vi "TwoCameraDisplayPanel.vi"() -> ()   [LabVIEW 2011]
uses:
  MvLVLib/MvCameraControl.lvlib
  MvLVLib/VIs/CreateGigEHandle.vi
  MvLVLib/VIs/CreateU3VHandle.vi
  <vilib>/picture/picture.llb/imagedata.ctl
panel:
  in  "image data 2":T1 caption="图像数据"
  in  "Rectangle 2":T2
  out "pFrameInfoEx out 2":T3
  in  "pConvertInfo In 2":T4
  out "nWidth 2":u32
  out "nHeight 2":u32
  out "PayloadSize 2":u32
  out "PixelFormat 2":u32
  out "handle out 2":u64
  in  "handle 2":u64
  out "Picture 2":picture
  in  "Device List 2":u16(ring)
  out "U3VDeviceArray":T5(array[cluster])
  out "GigEDeviceArray":T6(array[cluster])
  in  "pConvertInfo In":T4
  out "PixelFormat":u32
  out "handle out":u64
  in  "handle":u64
  in  "Rectangle":T2
  in  "image data":T1 caption="图像数据"
  out "Picture":picture
  out "PayloadSize":u32
  out "pFrameInfoEx out":T3
  out "nHeight":u32
  out "nWidth":u32
  out "Acquisision Flag":bool
  in  "Trigger Mode":bool
  in  "Continuous":bool
  out "打开标志":bool
  in  "stop":bool
  in  "Trigger Once":bool
  in  "Stop":bool
  in  "Start":bool
  in  "Open Device":bool
  in  "Close Device":bool
  in  "error in (no error) 2":errorcluster caption="错误输入（无错误）"
  in  "Refresh Devices":bool
  in  "Device List":u16(ring)
  # "Initialize"
  # "Acquisition"
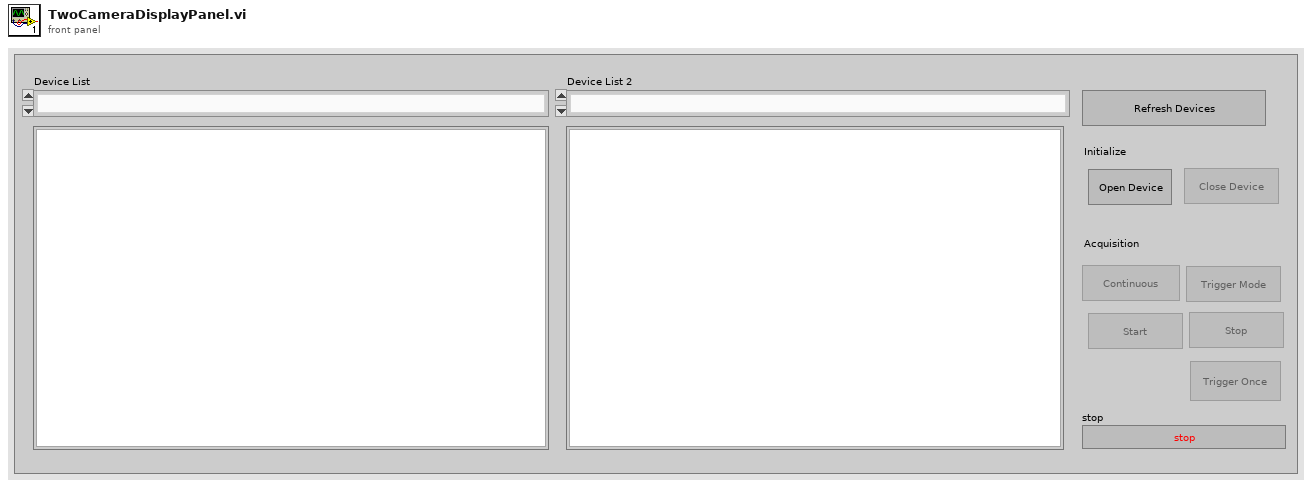
[diagram p1: front panel]
types:
  T1 = typedef "imagedata.ctl" = cluster{"image type":i32, "image depth":i32, "image":u8[], "mask":u8[], "colors":u32[], "Rectangle":cluster{"left":i16, "top":i16, "right":i16, "bottom":i16}}
  T2 = cluster{"left":i16, "top":i16, "right":i16, "bottom":i16}
  T3 = cluster{"nWidth":u16, "nHeight":u16, "enPixelType":i32, "nFrameNum":u32, "nDevTimeStampHigh":u32, "nDevTimeStampLow":u32, "nReserved0":u32, "nHostTimeStamp":i64, "nFrameLen":u32, "nSecondCount]":u32, "nCycleCount":u32, "nCycleOffset":u32, "fGain":u32, "fExposureTime":u32, "nAverageBrightness":u32, "nRed":u32, "nGreen":u32, "nBlue":u32, "nFrameCounter":u32, "nTriggerIndex":u32, "nInput":u32, "nOutput":u32, "nOffsetX":u32, "nOffsetY":u32, "nReserved[0]":u32, "nReserved[1]":u32, "nReserved[2]":u32, "nReserved[3]":u32, "nReserved[4]":u32, "nReserved[5]":u32, "nReserved[6]":u32, "nReserved[7]":u32, "nReserved[8]":u32, "nReserved[9]":u32, "nReserved[10]":u32, "nReserved[11]":u32, "nReserved[12]":u32, "nReserved[13]":u32, "nReserved[14] 10":u32, "nReserved[15] 11":u32, "nReserved[16] 12":u32, "nReserved[17] 13":u32, "nReserved[18] 14":u32, "nReserved[19] 15":u32, "nReserved[20] 16":u32, "nReserved[21] 17":u32, "nReserved[22] 18":u32, "nReserved[23] 19":u32, "nReserved[24] 20":u32, "nReserved[25] 21":u32, "nReserved[26] 22":u32, "nReserved[27] 23":u32, "nReserved[28] 24":u32, "nReserved[29] 25":u32, "nReserved[30] 26":u32, "nReserved[31] 27":u32, "nReserved[32] 28":u32, "nReserved[33] 29":u32, "nReserved[34] 30":u32, "nReserved[35] 31":u32, "nReserved[36] 32":u32, "nReserved[37] 33":u32, "nReserved[38] 34":u32, "nReserved[39] 35":u32, "nReserved[40] 36":u32}
  T4 = cluster{"nWidth":u16, "nHeight":u16, "enSrcPixelType":u32, "nSrcDataLen":u32, "enDstPixelType":u32, "nDstLen":u32, "nDstBufferSize":u32, "nRes0":u32, "nRes1":u32, "nRes2":u32, "nRes3":u32}
  T5 = cluster{"nMajorVer":u16, "nMinorVer":u16, "nMacAddrHigh":u32, "nMacAddrLow":u32, "nTLayerType":u32, "nReserved0":u32, "nReserved1":u32, "nReserved2":u32, "nReserved3":u32, "CrtlInEndPoint":u8, "CrtlOutEndPoint":u8, "StreamEndPoint":u8, "EventEndPoint":u8, "idVendor":u16, "idProduct":u16, "nDeviceNumber":u32, "nRes0":u32, "nRes1":u32, "chDeviceGUID":string, "chVendorName":string, "chModelName":string, "chFamilyName":string, "chDeviceVersion":string, "chManufacturerName":string, "chSerialNumber":string, "chUserDefinedName":string, "nbcdUSB":u32, "nRes2":u32, "nRes3":u32}[]
  T6 = cluster{"nMajorVer":u16, "nMinorVer":u16, "nMacAddrHigh":u32, "nMacAddrLow":u32, "nTLayerType":u32, "nReserved0":u32, "nReserved1":u32, "nReserved2":u32, "nReserved3":u32, "nIpCfgOption":u32, "nIpCfgCurrent":u32, "nCurrentIp":u32, "nCurrentSubNetMask":u32, "nDefaultGateWay":u32, "chManualfacturerName":string, "chModelName":string, "chDeviceVersion":string, "chManufacturerSpecificInfo":string, "chSerialNumber":string, "chUserDefinedName":string, "nRes0":string, "nRes1":string, "nNetExport":u32, "nRes2":u32, "nRes3":u32}[]
  T7 = enum8{"Enabled", "Disabled", "Disabled and Grayed Out"}
  T8 = cluster{"nCurValue":u32, "nMax":u32, "nMin":u32, "nInc":u32, "nReserved[0]":u32, "nReserved[1]":u32, "nReserved[2]":u32, "nReserved[3]":u32}
  T9 = cluster{"nCurValue":u32, "nSupportedNum":u32, "nSupportValue[0]":u32, "nSupportValue[1]":u32, "nSupportValue[2]":u32, "nSupportValue[3]":u32, "nSupportValue[4]":u32, "nSupportValue[5]":u32, "nSupportValue[6]":u32, "nSupportValue[7]":u32, "nSupportValue[8]":u32, "nSupportValue[9]":u32, "nSupportValue[10]":u32, "nSupportValue[11]":u32, "nSupportValue[12]":u32, "nSupportValue[13]":u32, "nSupportValue[14]":u32, "nSupportValue[15]":u32, "nSupportValue[16]":u32, "nSupportValue[17]":u32, "nSupportValue[18]":u32, "nSupportValue[19]":u32, "nSupportValue[20]":u32, "nSupportValue[21]":u32, "nSupportValue[22]":u32, "nSupportValue[23]":u32, "nSupportValue[24]":u32, "nSupportValue[25]":u32, "nSupportValue[26]":u32, "nSupportValue[27]":u32, "nSupportValue[28]":u32, "nSupportValue[29]":u32, "nSupportValue[30]":u32, "nSupportValue[31]":u32, "nSupportValue[32]":u32, "nSupportValue[33]":u32, "nSupportValue[34]":u32, "nSupportValue[35]":u32, "nSupportValue[36]":u32, "nSupportValue[37]":u32, "nSupportValue[38]":u32, "nSupportValue[39]":u32, "nSupportValue[40]":u32, "nSupportValue[41]":u32, "nSupportValue[42]":u32, "nSupportValue[43]":u32, "nSupportValue[44]":u32, "nSupportValue[45]":u32, "nSupportValue[46]":u32, "nSupportValue[47]":u32, "nSupportValue[48]":u32, "nSupportValue[49]":u32, "nSupportValue[50]":u32, "nSupportValue[51]":u32, "nSupportValue[52]":u32, "nSupportValue[53]":u32, "nSupportValue[54]":u32, "nSupportValue[55]":u32, "nSupportValue[56]":u32, "nSupportValue[57]":u32, "nSupportValue[58]":u32, "nSupportValue[59]":u32, "nSupportValue[60]":u32, "nSupportValue[61]":u32, "nSupportValue[62]":u32, "nSupportValue[63]":u32, "nReserved[0]":u32, "nReserved[1]":u32, "nReserved[2]":u32, "nReserved[3]":u32}
  T10 = cluster{"nMajorVer":u16, "nMinorVer":u16, "nMacAddrHigh":u32, "nMacAddrLow":u32, "nTLayerType":u32, "nReserved0":u32, "nReserved1":u32, "nReserved2":u32, "nReserved3":u32, "CrtlInEndPoint":u8, "CrtlOutEndPoint":u8, "StreamEndPoint":u8, "EventEndPoint":u8, "idVendor":u16, "idProduct":u16, "nDeviceNumber":u32, "nRes0":u32, "nRes1":u32, "chDeviceGUID":string, "chVendorName":string, "chModelName":string, "chFamilyName":string, "chDeviceVersion":string, "chManufacturerName":string, "chSerialNumber":string, "chUserDefinedName":string, "nbcdUSB":u32, "nRes2":u32, "nRes3":u32}
  T11 = cluster{"nMajorVer":u16, "nMinorVer":u16, "nMacAddrHigh":u32, "nMacAddrLow":u32, "nTLayerType":u32, "nReserved0":u32, "nReserved1":u32, "nReserved2":u32, "nReserved3":u32, "nIpCfgOption":u32, "nIpCfgCurrent":u32, "nCurrentIp":u32, "nCurrentSubNetMask":u32, "nDefaultGateWay":u32, "chManualfacturerName":string, "chModelName":string, "chDeviceVersion":string, "chManufacturerSpecificInfo":string, "chSerialNumber":string, "chUserDefinedName":string, "nRes0":string, "nRes1":string, "nNetExport":u32, "nRes2":u32, "nRes3":u32}
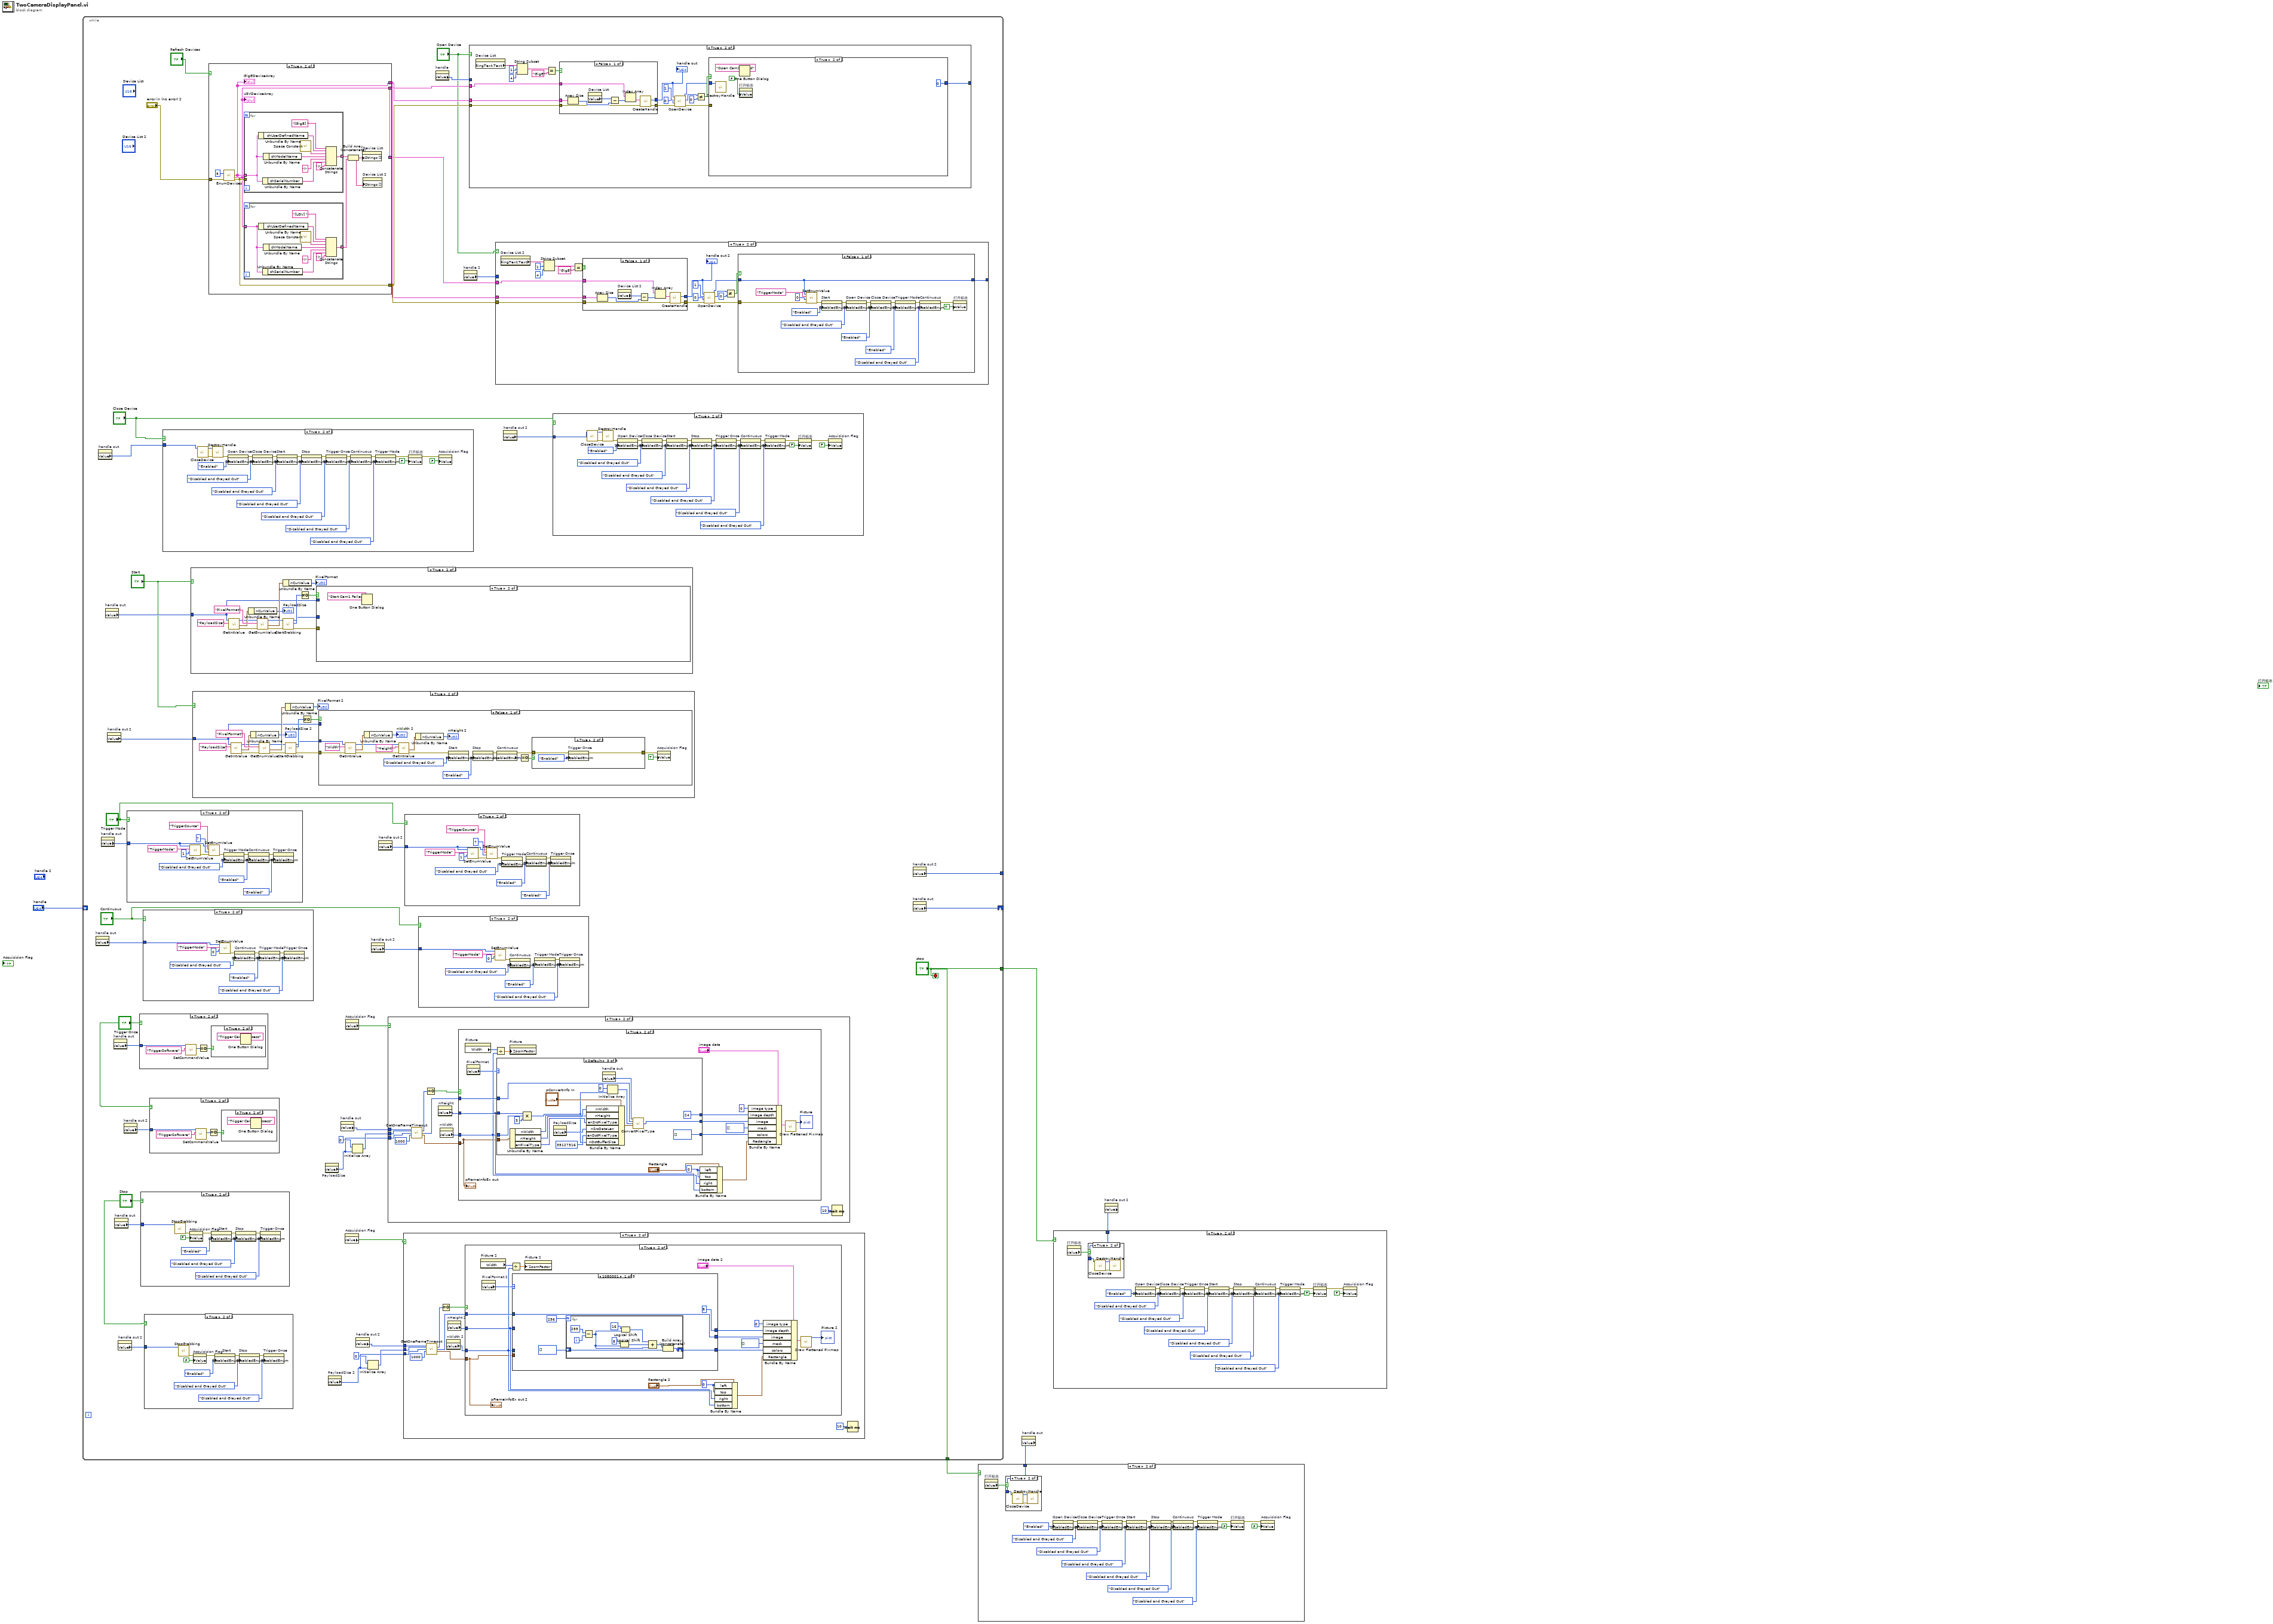
[diagram p0: block diagram]
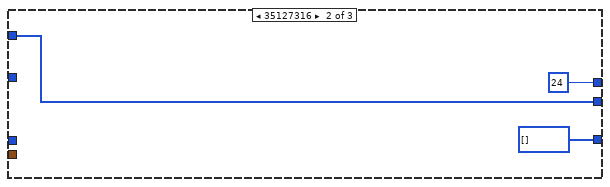
[diagram p8: hidden frame]
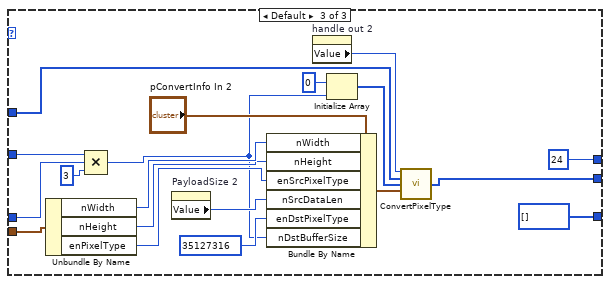
[diagram p9: hidden frame]
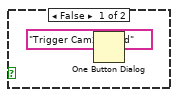
[diagram p11: hidden frame]
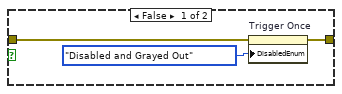
[diagram p16: hidden frame]
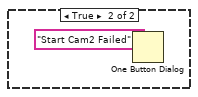
[diagram p17: hidden frame]
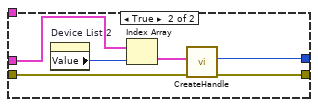
[diagram p20: hidden frame]
diagram:
  n1 = while {
    tunnel: ["stop"] -> w5
    shift-right: [w43] -> _
    shift-left: "handle" -> [_]
    tunnel: ["stop"] -> w1
    tunnel: [w9] -> _
    stop <- "stop" stop-if-true
    n2 = property on="handle out" class="DigNum (strict)"() -> ("Value"=w35:u64)  [unwired: 2 in, 2 out]
    n3 = property on="handle out" class="DigNum (strict)"() -> ("Value"=w41:u64)  [unwired: 2 in, 2 out]
    n4 = property on="handle out" class="DigNum (strict)"() -> ("Value"=w36:u64)  [unwired: 2 in, 2 out]
    n5 = property on="handle out" class="DigNum (strict)"() -> ("Value"=w37:u64)  [unwired: 2 in, 2 out]
    n6 = property on="handle out 2" class="DigNum (strict)"() -> ("Value"=w23:u64)  [unwired: 2 in, 2 out]
    n7 = property on="handle out" class="DigNum (strict)"() -> ("Value"=w40:u64)  [unwired: 2 in, 2 out]
    n8 = property on="handle out" class="DigNum (strict)"() -> ("Value"=w39:u64)  [unwired: 2 in, 2 out]
    n9 = property on="handle out 2" class="DigNum (strict)"() -> ("Value"=w17:u64)  [unwired: 2 in, 2 out]
    n10 = property on="handle out 2" class="DigNum (strict)"() -> ("Value"=w16:u64)  [unwired: 2 in, 2 out]
    n11 = case shown="True" "Trigger Mode" {
      tunnel: w36 -> [_ w347]
      frame False {
      }
      frame True {
        n12 = call "SetEnumValue.vi"("nValue"=u32 1, "strKey"="TriggerMode", "handle"=w347) -> ("error out"=w353:errorcluster)  [unwired: 6 in, 2 out]
        n13 = call "SetEnumValue.vi"("error in (no error)"=w353, "nValue"=u32 7, "strKey"="TriggerSource", "handle"=w347) -> ("error out"=w352:errorcluster)  [unwired: 5 in, 2 out]
        n14 = property on="Trigger Mode" class="Bool"(error in=w352, "DisabledEnum"=T7."Disabled and Grayed Out" ("禁用")) -> (error out=w351:errorcluster)  [unwired: 1 in, 1 out]
        n15 = property on="Continuous" class="Bool"(error in=w351, "DisabledEnum"=T7."Enabled" ("禁用")) -> (error out=w349:errorcluster)  [unwired: 1 in, 1 out]
        n16 = property on="Trigger Once" class="Bool"(error in=w349, "DisabledEnum"=T7."Enabled" ("禁用")) -> ()  [unwired: 1 in, 2 out]
      }
    }
    n17 = case shown="True" "Trigger Once" {
      tunnel: w40 -> [_ w362]
      frame False {
      }
      frame True {
        n18 = call "SetCommandValue.vi"("strValue"="TriggerSoftware", "handle"=w362) -> ("function return"=w360:i32)  [unwired: 7 in, 2 out]
        n19 = Equal To 0?(x=w360) -> (x = 0?=w359:bool)
        n20 = case shown="True" w359 {
          frame False {
            n21 = One Button Dialog(message="Trigger Cam1 Failed") -> ()  [unwired: 1 in, 1 out]
          }
          frame True {
            n22 = One Button Dialog(message="Trigger Can1 Success") -> ()  [unwired: 1 in, 1 out]
          }
        }
      }
    }
    n23 = case shown="True" "Stop" {
      tunnel: w39 -> [_ w337]
      frame False {
      }
      frame True {
        n24 = call "StopGrabbing.vi"("handle"=w337) -> ("error out"=w336:errorcluster)  [unwired: 8 in, 2 out]
        n25 = property on="Acquisision Flag" class="Bool (strict)"(error in=w336, "Value"=FALSE ("采集标志")) -> (error out=w331:errorcluster)  [unwired: 1 in, 1 out]
        n26 = property on="Start" class="Bool"(error in=w331, "DisabledEnum"=T7."Enabled" ("禁用")) -> (error out=w330:errorcluster)  [unwired: 1 in, 1 out]
        n27 = property on="Stop" class="Bool"(error in=w330, "DisabledEnum"=T7."Disabled and Grayed Out" ("禁用")) -> (error out=w329:errorcluster)  [unwired: 1 in, 1 out]
        n28 = property on="Trigger Once" class="Bool"(error in=w329, "DisabledEnum"=T7."Disabled and Grayed Out" ("禁用")) -> ()  [unwired: 1 in, 2 out]
      }
    }
    n29 = case shown="True" "Continuous" {
      tunnel: w35 -> [_ w338]
      frame False {
      }
      frame True {
        n30 = call "SetEnumValue.vi"("nValue"=u32 0, "strKey"="TriggerMode", "handle"=w338) -> ("error out"=w339:errorcluster)  [unwired: 6 in, 2 out]
        n31 = property on="Continuous" class="Bool"(error in=w339, "DisabledEnum"=T7."Disabled and Grayed Out" ("禁用")) -> (error out=w343:errorcluster)  [unwired: 1 in, 1 out]
        n32 = property on="Trigger Mode" class="Bool"(error in=w343, "DisabledEnum"=T7."Enabled" ("禁用")) -> (error out=w341:errorcluster)  [unwired: 1 in, 1 out]
        n33 = property on="Trigger Once" class="Bool"(error in=w341, "DisabledEnum"=T7."Disabled and Grayed Out" ("禁用")) -> ()  [unwired: 1 in, 2 out]
      }
    }
    n34 = case shown="True" "Stop" {
      tunnel: w17 -> [_ w126]
      frame False {
      }
      frame True {
        n35 = call "StopGrabbing.vi"("handle"=w126) -> ("error out"=w125:errorcluster)  [unwired: 8 in, 2 out]
        n36 = property on="Acquisision Flag" class="Bool (strict)"(error in=w125, "Value"=FALSE ("采集标志")) -> (error out=w120:errorcluster)  [unwired: 1 in, 1 out]
        n37 = property on="Start" class="Bool"(error in=w120, "DisabledEnum"=T7."Enabled" ("禁用")) -> (error out=w119:errorcluster)  [unwired: 1 in, 1 out]
        n38 = property on="Stop" class="Bool"(error in=w119, "DisabledEnum"=T7."Disabled and Grayed Out" ("禁用")) -> (error out=w118:errorcluster)  [unwired: 1 in, 1 out]
        n39 = property on="Trigger Once" class="Bool"(error in=w118, "DisabledEnum"=T7."Disabled and Grayed Out" ("禁用")) -> ()  [unwired: 1 in, 2 out]
      }
    }
    n40 = case shown="True" "Trigger Once" {
      tunnel: w16 -> [_ w115]
      frame False {
      }
      frame True {
        n41 = call "SetCommandValue.vi"("strValue"="TriggerSoftware", "handle"=w115) -> ("function return"=w113:i32)  [unwired: 7 in, 2 out]
        n42 = Equal To 0?(x=w113) -> (x = 0?=w112:bool)
        n43 = case shown="True" w112 {
          frame False {
            n44 = One Button Dialog(message="Trigger Cam2 Failed") -> ()  [unwired: 1 in, 1 out]
          }
          frame True {
            n45 = One Button Dialog(message="Trigger Cam2 Success") -> ()  [unwired: 1 in, 1 out]
          }
        }
      }
    }
    n46 = case shown="True" "Close Device" {
      tunnel: w41 -> [_ w408]
      frame False {
      }
      frame True {
        n47 = call "CloseDevice.vi"("handle"=w408) -> ("error out"=w410:errorcluster, "handle out"=w407:u64)  [unwired: 8 in, 1 out]
        n48 = call "DestroyHandle.vi"("error in (no error)"=w410, "handle"=w407) -> ("error out"=w409:errorcluster)  [unwired: 8 in, 1 out]
        n49 = property on="Open Device" class="Bool"(error in=w409, "DisabledEnum"=T7."Enabled" ("禁用")) -> (error out=w423:errorcluster)  [unwired: 1 in, 1 out]
        n50 = property on="Close Device" class="Bool"(error in=w423, "DisabledEnum"=T7."Disabled and Grayed Out" ("禁用")) -> (error out=w422:errorcluster)  [unwired: 1 in, 1 out]
        n51 = property on="Start" class="Bool"(error in=w422, "DisabledEnum"=T7."Disabled and Grayed Out" ("禁用")) -> (error out=w421:errorcluster)  [unwired: 1 in, 1 out]
        n52 = property on="Stop" class="Bool"(error in=w421, "DisabledEnum"=T7."Disabled and Grayed Out" ("禁用")) -> (error out=w420:errorcluster)  [unwired: 1 in, 1 out]
        n53 = property on="Trigger Once" class="Bool"(error in=w420, "DisabledEnum"=T7."Disabled and Grayed Out" ("禁用")) -> (error out=w417:errorcluster)  [unwired: 1 in, 1 out]
        n54 = property on="Continuous" class="Bool"(error in=w417, "DisabledEnum"=T7."Disabled and Grayed Out" ("禁用")) -> (error out=w415:errorcluster)  [unwired: 1 in, 1 out]
        n55 = property on="Trigger Mode" class="Bool"(error in=w415, "DisabledEnum"=T7."Disabled and Grayed Out" ("禁用")) -> (error out=w414:errorcluster)  [unwired: 1 in, 1 out]
        n56 = property on="打开标志" class="Bool (strict)"(error in=w414, "Value"=FALSE ("打开标志")) -> (error out=w412:errorcluster)  [unwired: 1 in, 1 out]
        n57 = property on="Acquisision Flag" class="Bool (strict)"(error in=w412, "Value"=FALSE ("采集标志")) -> ()  [unwired: 1 in, 2 out]
      }
    }
    n58 = case shown="True" "Start" {
      tunnel: w37 -> [_ w369]
      frame False {
      }
      frame True {
        n59 = call "GetIntValue.vi"("strKey"="PayloadSize", "handle"=w369) -> ("error out"=w375:errorcluster, "pIntValue out"=w371:T8, "handle out"=w367:u64)  [unwired: 6 in, 1 out]
        n60 = Unbundle By Name(w371) -> ("nCurValue"=→"PayloadSize":u32)
        n61 = call "GetEnumValue.vi"("error in (no error)"=w375, "strKey"="PixelFormat", "handle"=w367) -> ("error out"=w374:errorcluster, "pEnumValue out"=w376:T9, "handle out"=w366:u64)  [unwired: 5 in, 1 out]
        n62 = Unbundle By Name(w376) -> ("nCurValue"=→"PixelFormat":u32)
        n63 = call "StartGrabbing.vi"("error in (no error)"=w374, "handle"=w366) -> ("error out"=w373:errorcluster, "function return"=w379:i32, "handle out"=w365:u64)  [unwired: 7 in]
        n64 = Not Equal To 0?(x=w379) -> (x != 0?=w378:bool)
        n65 = case shown="True" w378 {
          tunnel: w369 -> [_ _]
          tunnel: w373 -> [w382 _]
          tunnel: w365 -> [w381 _]
          frame False {
            n66 = call "GetIntValue.vi"("error in (no error)"=w382, "strKey"="Width", "handle"=w381) -> ("error out"=w389:errorcluster, "pIntValue out"=w383:T8, "handle out"=w380:u64)  [unwired: 5 in, 1 out]
            n67 = Unbundle By Name(w383) -> ("nCurValue"=→"nWidth":u32)
            n68 = call "GetIntValue.vi"("error in (no error)"=w389, "strKey"="Height", "handle"=w380) -> ("error out"=w388:errorcluster, "pIntValue out"=w386:T8)  [unwired: 5 in, 2 out]
            n69 = Unbundle By Name(w386) -> ("nCurValue"=→"nHeight":u32)
            n70 = property on="Start" class="Bool"(error in=w388, "DisabledEnum"=T7."Disabled and Grayed Out" ("禁用")) -> (error out=w398:errorcluster)  [unwired: 1 in, 1 out]
            n71 = property on="Stop" class="Bool"(error in=w398, "DisabledEnum"=T7."Enabled" ("禁用")) -> (error out=w384:errorcluster)  [unwired: 1 in, 1 out]
            n72 = property on="Continuous" class="Bool"(error in=w384) -> (error out=w394:errorcluster, "DisabledEnum"=w395:T7)  [unwired: 1 in, 1 out]
            n73 = Equal To 0?(x=w395) -> (x = 0?=w396:bool)
            n74 = case shown="True" w396 {
              tunnel: w394 -> [w401 w404]
              tunnel: [w400 w403] -> w393
              frame False {
                n75 = property on="Trigger Once" class="Bool"(error in=w401, "DisabledEnum"=T7."Disabled and Grayed Out" ("禁用")) -> (error out=w400:errorcluster)  [unwired: 1 in, 1 out]
              }
              frame True {
                n76 = property on="Trigger Once" class="Bool"(error in=w404, "DisabledEnum"=T7."Enabled" ("禁用")) -> (error out=w403:errorcluster)  [unwired: 1 in, 1 out]
              }
            }
            n77 = property on="Acquisision Flag" class="Bool (strict)"(error in=w393, "Value"=TRUE ("采集标志")) -> ()  [unwired: 1 in, 2 out]
          }
          frame True {
            n78 = One Button Dialog(message="Start Cam1 Failed") -> ()  [unwired: 1 in, 1 out]
          }
        }
      }
    }
    n79 = case shown="True" "Start" {
      tunnel: w23 -> [_ w150]
      frame False {
      }
      frame True {
        n80 = call "GetIntValue.vi"("strKey"="PayloadSize", "handle"=w150) -> ("error out"=w156:errorcluster, "pIntValue out"=w152:T8, "handle out"=w148:u64)  [unwired: 6 in, 1 out]
        n81 = Unbundle By Name(w152) -> ("nCurValue"=→"PayloadSize 2":u32)
        n82 = call "GetEnumValue.vi"("error in (no error)"=w156, "strKey"="PixelFormat", "handle"=w148) -> ("error out"=w155:errorcluster, "pEnumValue out"=w157:T9, "handle out"=w147:u64)  [unwired: 5 in, 1 out]
        n83 = Unbundle By Name(w157) -> ("nCurValue"=→"PixelFormat 2":u32)
        n84 = call "StartGrabbing.vi"("error in (no error)"=w155, "handle"=w147) -> ("error out"=w154:errorcluster, "function return"=w160:i32, "handle out"=w146:u64)  [unwired: 7 in]
        n85 = Not Equal To 0?(x=w160) -> (x != 0?=w159:bool)
        n86 = case shown="False" w159 {
          tunnel: w150 -> [_ _]
          tunnel: w154 -> [w165 _]
          tunnel: w146 -> [w164 _]
          frame False {
            n87 = call "GetIntValue.vi"("error in (no error)"=w165, "strKey"="Width", "handle"=w164) -> ("error out"=w171:errorcluster, "pIntValue out"=w166:T8, "handle out"=w163:u64)  [unwired: 5 in, 1 out]
            n88 = Unbundle By Name(w166) -> ("nCurValue"=→"nWidth 2":u32)
            n89 = call "GetIntValue.vi"("error in (no error)"=w171, "strKey"="Height", "handle"=w163) -> ("error out"=w162:errorcluster, "pIntValue out"=w169:T8)  [unwired: 5 in, 2 out]
            n90 = Unbundle By Name(w169) -> ("nCurValue"=→"nHeight 2":u32)
            n91 = property on="Start" class="Bool"(error in=w162, "DisabledEnum"=T7."Disabled and Grayed Out" ("禁用")) -> ()  [unwired: 1 in, 2 out]
            n92 = property on="Stop" class="Bool"("DisabledEnum"=T7."Enabled" ("禁用")) -> (error out=w167:errorcluster)  [unwired: 2 in, 1 out]
            n93 = property on="Continuous" class="Bool"(error in=w167) -> (error out=w176:errorcluster, "DisabledEnum"=w177:T7)  [unwired: 1 in, 1 out]
            n94 = Equal To 0?(x=w177) -> (x = 0?=w178:bool)
            n95 = case shown="True" w178 {
              tunnel: w176 -> [w181 w184]
              tunnel: [w180 w183] -> w175
              frame False {
                n96 = property on="Trigger Once" class="Bool"(error in=w181, "DisabledEnum"=T7."Disabled and Grayed Out" ("禁用")) -> (error out=w180:errorcluster)  [unwired: 1 in, 1 out]
              }
              frame True {
                n97 = property on="Trigger Once" class="Bool"(error in=w184, "DisabledEnum"=T7."Enabled" ("禁用")) -> (error out=w183:errorcluster)  [unwired: 1 in, 1 out]
              }
            }
            n98 = property on="Acquisision Flag" class="Bool (strict)"(error in=w175, "Value"=TRUE ("采集标志")) -> ()  [unwired: 1 in, 2 out]
          }
          frame True {
            n99 = One Button Dialog(message="Start Cam2 Failed") -> ()  [unwired: 1 in, 1 out]
          }
        }
      }
    }
    n100 = case shown="True" "Refresh Devices" {
      tunnel: [w485 w492] -> w30
      tunnel: "error in (no error) 2" -> [w485 w491]
      tunnel: [w483 w486] -> w31
      tunnel: [w484 w488] -> w29
      tunnel: [w483 w486] -> w28
      frame False {
        n101 = property on="U3VDeviceArray" class="Arr (strict)"() -> ("Value"=w483:T5)  [unwired: 2 in, 2 out]
        n102 = property on="GigEDeviceArray" class="Arr (strict)"() -> ("Value"=w484:T6)  [unwired: 2 in, 2 out]
      }
      frame True {
        n103 = call "EnumDevices.vi"("nLayerType"=u32 5, "error in (no error)"=w491) -> ("GigEDeviceArray"=w488:T6, "U3VDeviceArray"=w486:T5, "error out"=w492:errorcluster)  [unwired: 9 in, 2 out]
        "GigEDeviceArray" <- w488
        "U3VDeviceArray" <- w486
        n104 = for {
          tunnel: w492 -> [_]
          tunnel: w488 -> [w505] mode=indexing
          tunnel: [w504] -> w490 mode=indexing
          n105 = Unbundle By Name(w505) -> ("chUserDefinedName"=w508:string)
          n106 = Unbundle By Name(w505) -> ("chSerialNumber"=w506:string)
          n107 = Unbundle By Name(w505) -> ("chModelName"=w507:string)
          n108 = call <vilib>:"Space Constant.vi"() -> ("String"=w511:string)
          n109 = Concatenate Strings("[GigE] " ("字符串"), w508, w511, w507, "(" ("字符串"), w506, ")" ("字符串")) -> (w504:string)
        }
        n110 = for {
          tunnel: w486 -> [w498] mode=indexing
          tunnel: [w495] -> w489 mode=indexing
          n111 = Unbundle By Name(w498) -> ("chUserDefinedName"=w502:string)
          n112 = Unbundle By Name(w498) -> ("chSerialNumber"=w497:string)
          n113 = Unbundle By Name(w498) -> ("chModelName"=w500:string)
          n114 = call <vilib>:"Space Constant.vi"() -> ("String"=w501:string)
          n115 = Concatenate Strings("[U3V] " ("字符串"), w502, w501, w500, "(" ("字符串"), w497, ")" ("字符串")) -> (w495:string)
        }
        n116 = Build Array (concatenate)(w490, w489) -> (w487:string[])
        n117 = property on="Device List" class="Ring (strict)"("Strings []"=w487) -> ()  [unwired: 2 in, 2 out]
        n118 = property on="Device List 2" class="Ring (strict)"("Strings []"=w487) -> ()  [unwired: 2 in, 2 out]
      }
    }
    n119 = property on="PayloadSize" class="DigNum (strict)"() -> ("Value"=w32:u32)  [unwired: 2 in, 2 out]
    n120 = property on="PayloadSize 2" class="DigNum (strict)"() -> ("Value"=w11:u32)  [unwired: 2 in, 2 out]
    n121 = property on="handle out" class="DigNum (strict)"() -> ("Value"=w38:u64)  [unwired: 2 in, 2 out]
    n122 = property on="Acquisision Flag" class="Bool (strict)"() -> ("Value"=w7:bool)  [unwired: 2 in, 2 out]
    n123 = property on="Acquisision Flag" class="Bool (strict)"() -> ("Value"=w8:bool)  [unwired: 2 in, 2 out]
    n124 = Initialize Array(u8 0 ("元素"), w32) -> (w33:u8[])
    n125 = property on="handle out 2" class="DigNum (strict)"() -> ("Value"=w14:u64)  [unwired: 2 in, 2 out]
    n126 = Initialize Array(u8 0 ("元素"), w11) -> (w12:u8[])
    n127 = property on="handle out 2" class="DigNum (strict)"() -> ("Value"=w19:u64)  [unwired: 2 in, 2 out]
    n128 = property on="handle out 2" class="DigNum (strict)"() -> ("Value"=w21:u64)  [unwired: 2 in, 2 out]
    n129 = case shown="True" w8 {
      tunnel: w38 -> [_ w268]
      tunnel: w33 -> [_ w267]
      tunnel: w32 -> [_ w266]
      frame False {
      }
      frame True {
        n130 = call "GetOneFrameTimeout.vi"("handle"=w268, "pData"=w267, "nDataSize"=w266, "nMsec"=1000) -> ("function return"=w265:i32, "pData Out"=w264:u8[], "pFrameInfoEx out"=w263:T3)  [unwired: 7 in, 2 out]
        n131 = Equal To 0?(x=w265) -> (x = 0?=w272:bool)
        n132 = property on="nHeight" class="DigNum (strict)"() -> ("Value"=w270:u32)  [unwired: 2 in, 2 out]
        n133 = property on="nWidth" class="DigNum (strict)"() -> ("Value"=w271:u32)  [unwired: 2 in, 2 out]
        n134 = case shown="True" w272 {
          tunnel: w264 -> [_ w281]
          tunnel: w271 -> [_ w279]
          tunnel: w270 -> [_ w280]
          tunnel: w263 -> [_ w275]
          frame False {
          }
          frame True {
            w288 = i16 0 ("left")
            n135 = property on="Picture" class="Pict"() -> ("Width"=w283:u32)  [unwired: 2 in, 2 out]
            n136 = property on="PixelFormat" class="DigNum (strict)"() -> ("Value"=w276:u32)  [unwired: 2 in, 2 out]
            n137 = Divide(x=w283, y=w279) -> (x/y=w282:dbl)
            n138 = case shown="Default" w276 {
              tunnel: w281 -> [w294 w309 w325]
              tunnel: w280 -> [_ _ w322]
              tunnel: w279 -> [_ _ w321]
              tunnel: [w294 w309 w310] -> w278
              tunnel: [8 24 24] -> w274
              tunnel: [w292 i32[] [] i32[] []] -> w277
              tunnel: w275 -> [_ _ w311]
              frame 17301505 {
                n139 = for {
                  N: 256 -> [_]
                  shift-right: [w301] -> w292
                  shift-left: i32[] [] ("数组") -> [w300]
                  i -> [w297]
                  n140 = Subtract(x=255, y=w297) -> (x-y=w298:i32)
                  n141 = Logical Shift(y=i16 8, x=w298) -> (x << y=w303:i32)
                  n142 = Logical Shift(y=16 ("x"), x=w298) -> (x << y=w304:i32)
                  n143 = Compound Arithmetic op=ADD(w304, w303, w298) -> (w302:i32)
                  n144 = Build Array (concatenate)(w302, w300) -> (w301:i32[])
                }
              }
              frame 35127316 {
              }
              frame Default {
                n145 = Unbundle By Name(w311) -> ("nWidth"=w320:u16, "nHeight"=w319:u16, "enPixelType"=w318:i32)
                n146 = Compound Arithmetic op=MULTIPLY(w322, w321, u32 3 ("值")) -> (w315:u32)
                n147 = property on="PayloadSize" class="DigNum (strict)"() -> ("Value"=w317:u32)  [unwired: 2 in, 2 out]
                n148 = Bundle By Name(cluster="pConvertInfo In", "nWidth"=w320, "nHeight"=w319, "enSrcPixelType"=w318, "nSrcDataLen"=w317, "enDstPixelType"=u32 35127316, "nDstBufferSize"=w315) -> (w314:T4)
                n149 = property on="handle out" class="DigNum (strict)"() -> ("Value"=w326:u64)  [unwired: 2 in, 2 out]
                n150 = Initialize Array(u8 0 ("元素"), w315) -> (w324:u8[])
                n151 = call "ConvertPixelType.vi"("handle"=w326, "pSrcData"=w325, "pDstBuf In"=w324, "pConvertInfo In"=w314) -> ("pDstBuf Out"=w310:u8[])  [unwired: 7 in, 4 out]
              }
            }
            n152 = property on="Picture" class="Pict"("ZoomFactor"=w282) -> ()  [unwired: 2 in, 2 out]
            n153 = Bundle By Name(cluster="Rectangle", "left"=w288, "top"=w288, "right"=w279, "bottom"=w280) -> (w285:T2)
            n154 = Bundle By Name(cluster="image data", "image type"=0, "image depth"=w274, "image"=w278, "mask"=u8[] [], "colors"=w277, "Rectangle"=w285) -> (w284:T1)
            n155 = call <vilib>:"Draw Flattened Pixmap.vi"("image data"=w284) -> ("new picture"=→"Picture":picture)  [unwired: 8 in]
            "pFrameInfoEx out" <- w275
          }
        }
        n156 = Wait (ms)(milliseconds to wait=u32 10 ("等待时间（毫秒）")) -> ()  [unwired: 1 out]
      }
    }
    n157 = case shown="True" w7 {
      tunnel: w14 -> [_ w51]
      tunnel: w12 -> [_ w50]
      tunnel: w11 -> [_ w49]
      frame False {
      }
      frame True {
        n158 = call "GetOneFrameTimeout.vi"("handle"=w51, "pData"=w50, "nDataSize"=w49, "nMsec"=1000) -> ("function return"=w48:i32, "pData Out"=w47:u8[], "pFrameInfoEx out"=w46:T3)  [unwired: 7 in, 2 out]
        n159 = Equal To 0?(x=w48) -> (x = 0?=w55:bool)
        n160 = property on="nWidth 2" class="DigNum (strict)"() -> ("Value"=w54:u32)  [unwired: 2 in, 2 out]
        n161 = property on="nHeight 2" class="DigNum (strict)"() -> ("Value"=w53:u32)  [unwired: 2 in, 2 out]
        n162 = case shown="True" w55 {
          tunnel: w47 -> [_ w67]
          tunnel: w54 -> [_ w65]
          tunnel: w53 -> [_ w66]
          tunnel: w46 -> [_ w60]
          frame False {
          }
          frame True {
            w74 = i16 0 ("left")
            n163 = property on="Picture 2" class="Pict"() -> ("Width"=w69:u32)  [unwired: 2 in, 2 out]
            n164 = property on="PixelFormat 2" class="DigNum (strict)"() -> ("Value"=w62:u32)  [unwired: 2 in, 2 out]
            n165 = Divide(x=w69, y=w65) -> (x/y=w68:dbl)
            n166 = case shown="1080001" w62 {
              tunnel: w67 -> [w77 w92 w108]
              tunnel: w66 -> [_ _ w105]
              tunnel: w65 -> [_ _ w104]
              tunnel: [w77 w92 w93] -> w64
              tunnel: [8 24 24] -> w57
              tunnel: [w75 i32[] [] i32[] []] -> w63
              tunnel: w60 -> [_ _ w94]
              frame 17301505 {
                n167 = for {
                  N: 256 -> [_]
                  shift-right: [w84] -> w75
                  shift-left: i32[] [] ("数组") -> [w83]
                  i -> [w80]
                  n168 = Subtract(x=255, y=w80) -> (x-y=w81:i32)
                  n169 = Logical Shift(y=i16 8, x=w81) -> (x << y=w86:i32)
                  n170 = Logical Shift(y=16 ("x"), x=w81) -> (x << y=w87:i32)
                  n171 = Compound Arithmetic op=ADD(w87, w86, w81) -> (w85:i32)
                  n172 = Build Array (concatenate)(w85, w83) -> (w84:i32[])
                }
              }
              frame 35127316 {
              }
              frame Default {
                n173 = Unbundle By Name(w94) -> ("nWidth"=w103:u16, "nHeight"=w102:u16, "enPixelType"=w101:i32)
                n174 = Compound Arithmetic op=MULTIPLY(w105, w104, u32 3 ("值")) -> (w98:u32)
                n175 = property on="PayloadSize 2" class="DigNum (strict)"() -> ("Value"=w100:u32)  [unwired: 2 in, 2 out]
                n176 = Bundle By Name(cluster="pConvertInfo In 2", "nWidth"=w103, "nHeight"=w102, "enSrcPixelType"=w101, "nSrcDataLen"=w100, "enDstPixelType"=u32 35127316, "nDstBufferSize"=w98) -> (w97:T4)
                n177 = property on="handle out 2" class="DigNum (strict)"() -> ("Value"=w109:u64)  [unwired: 2 in, 2 out]
                n178 = Initialize Array(u8 0 ("元素"), w98) -> (w107:u8[])
                n179 = call "ConvertPixelType.vi"("handle"=w109, "pSrcData"=w108, "pDstBuf In"=w107, "pConvertInfo In"=w97) -> ("pDstBuf Out"=w93:u8[])  [unwired: 7 in, 4 out]
              }
            }
            n180 = property on="Picture 2" class="Pict"("ZoomFactor"=w68) -> ()  [unwired: 2 in, 2 out]
            n181 = Bundle By Name(cluster="Rectangle 2", "left"=w74, "top"=w74, "right"=w65, "bottom"=w66) -> (w71:T2)
            n182 = Bundle By Name(cluster="image data 2", "image type"=0, "image depth"=w57, "image"=w64, "mask"=u8[] [], "colors"=w63, "Rectangle"=w71) -> (w70:T1)
            n183 = call <vilib>:"Draw Flattened Pixmap.vi"("image data"=w70) -> ("new picture"=→"Picture 2":picture)  [unwired: 8 in]
            "pFrameInfoEx out 2" <- w60
          }
        }
        n184 = Wait (ms)(milliseconds to wait=u32 10 ("等待时间（毫秒）")) -> ()  [unwired: 1 out]
      }
    }
    n185 = case shown="True" "Trigger Mode" {
      tunnel: w21 -> [_ w137]
      frame False {
      }
      frame True {
        n186 = call "SetEnumValue.vi"("nValue"=u32 1, "strKey"="TriggerMode", "handle"=w137) -> ("error out"=w141:errorcluster)  [unwired: 6 in, 2 out]
        n187 = call "SetEnumValue.vi"("error in (no error)"=w141, "nValue"=u32 7, "strKey"="TriggerSource", "handle"=w137) -> ("error out"=w136:errorcluster)  [unwired: 5 in, 2 out]
        n188 = property on="Trigger Mode" class="Bool"(error in=w136, "DisabledEnum"=T7."Disabled and Grayed Out" ("禁用")) -> ()  [unwired: 1 in, 2 out]
        n189 = property on="Continuous" class="Bool"("DisabledEnum"=T7."Enabled" ("禁用")) -> (error out=w139:errorcluster)  [unwired: 2 in, 1 out]
        n190 = property on="Trigger Once" class="Bool"(error in=w139, "DisabledEnum"=T7."Enabled" ("禁用")) -> ()  [unwired: 1 in, 2 out]
      }
    }
    n191 = case shown="True" "Continuous" {
      tunnel: w19 -> [_ w129]
      frame False {
      }
      frame True {
        n192 = call "SetEnumValue.vi"("nValue"=u32 0, "strKey"="TriggerMode", "handle"=w129) -> ("error out"=w128:errorcluster)  [unwired: 6 in, 2 out]
        n193 = property on="Continuous" class="Bool"(error in=w128, "DisabledEnum"=T7."Disabled and Grayed Out" ("禁用")) -> ()  [unwired: 1 in, 2 out]
        n194 = property on="Trigger Mode" class="Bool"("DisabledEnum"=T7."Enabled" ("禁用")) -> (error out=w131:errorcluster)  [unwired: 2 in, 1 out]
        n195 = property on="Trigger Once" class="Bool"(error in=w131, "DisabledEnum"=T7."Disabled and Grayed Out" ("禁用")) -> ()  [unwired: 1 in, 2 out]
      }
    }
    n196 = property on="handle" class="DigNum (strict)"() -> ("Value"=w42:u64)  [unwired: 2 in, 2 out]
    n197 = property on="handle 2" class="DigNum (strict)"() -> ("Value"=w27:u64)  [unwired: 2 in, 2 out]
    n198 = case shown="True" "Open Device" {
      tunnel: [w428 w440] -> _
      tunnel: w42 -> [w428 _]
      tunnel: w30 -> [_ w439]
      tunnel: w31 -> [_ w430]
      tunnel: w29 -> [_ w429]
      frame False {
      }
      frame True {
        n199 = property on="Device List" class="Ring (strict)"() -> ("RingText.Text"=w438:string)  [unwired: 2 in, 2 out]
        n200 = String Subset(string=w438, offset (0)=1 ("偏移量(0)"), length (rest)=4 ("长度（剩余）")) -> (substring=w435:string)
        n201 = Equal?(x=w435, y="GigE") -> (x = y?=w434:bool)
        n202 = case shown="False" w434 {
          tunnel: [w450 w459] -> w445
          tunnel: [w449 w458] -> w441
          tunnel: w429 -> [w454 w461]
          tunnel: w439 -> [w451 w460]
          tunnel: w430 -> [w456 _]
          frame False {
            n203 = Array Size(array=w454) -> (size(s)=w453:i32)
            n204 = property on="Device List" class="Ring (strict)"() -> ("Value"=w455:u16)  [unwired: 2 in, 2 out]
            n205 = Subtract(x=w455, y=w453) -> (x-y=w452:i32)
            n206 = Index Array(array=w456, index=w452) -> (element=w448:T10)
            n207 = call-poly "CreateHandle.vi"("error in (no error)"=w451, "U3VDevice"=w448) -> ("error out"=w450:errorcluster, "handle"=w449:u64)  [unwired: 6 in, 1 out]
          }
          frame True {
            n208 = property on="Device List" class="Ring (strict)"() -> ("Value"=w462:u16)  [unwired: 2 in, 2 out]
            n209 = Index Array(array=w461, index=w462) -> (element=w457:T11)
            n210 = call-poly "CreateHandle.vi"("error in (no error)"=w460, "GigEDevice"=w457) -> ("error out"=w459:errorcluster, "handle"=w458:u64)  [unwired: 6 in, 1 out]
          }
        }
        "handle out" <- w441
        n211 = call "OpenDevice.vi"("error in (no error)"=w445, "nSwitchoverKey"=u16 0, "nAccessMode"=u32 1, "handle"=w441) -> ("error out"=w442:errorcluster, "return"=w432:i32, "handle out"=w431:u64)  [unwired: 5 in]
        n212 = Not Equal?(x=w432, y=0) -> (x != y?=w446:bool)
        n213 = case shown="True" w446 {
          tunnel: w431 -> [w463 w480]
          tunnel: w442 -> [w464 _]
          tunnel: [w463 u64 0 ("handle")] -> w440
          frame False {
            n214 = call "SetEnumValue.vi"("error in (no error)"=w464, "nValue"=u32 0, "strKey"="TriggerMode", "handle"=w463) -> ("error out"=w475:errorcluster)  [unwired: 5 in, 2 out]
            n215 = property on="Start" class="Bool"(error in=w475, "DisabledEnum"=T7."Enabled" ("禁用")) -> (error out=w473:errorcluster)  [unwired: 1 in, 1 out]
            n216 = property on="Open Device" class="Bool"(error in=w473, "DisabledEnum"=T7."Disabled and Grayed Out" ("禁用")) -> (error out=w472:errorcluster)  [unwired: 1 in, 1 out]
            n217 = property on="Close Device" class="Bool"(error in=w472, "DisabledEnum"=T7."Enabled" ("禁用")) -> (error out=w469:errorcluster)  [unwired: 1 in, 1 out]
            n218 = property on="Trigger Mode" class="Bool"(error in=w469, "DisabledEnum"=T7."Enabled" ("禁用")) -> (error out=w467:errorcluster)  [unwired: 1 in, 1 out]
            n219 = property on="Continuous" class="Bool"(error in=w467, "DisabledEnum"=T7."Disabled and Grayed Out" ("禁用")) -> (error out=w465:errorcluster)  [unwired: 1 in, 1 out]
            n220 = property on="打开标志" class="Bool (strict)"(error in=w465, "Value"=TRUE ("布尔")) -> ()  [unwired: 1 in, 2 out]
          }
          frame True {
            n221 = call "DestroyHandle.vi"("handle"=w480) -> ()  [unwired: 9 in, 2 out]
            n222 = One Button Dialog(message="Open Cam1 Failed") -> ()  [unwired: 1 in, 1 out]
            n223 = property on="打开标志" class="Bool (strict)"("Value"=FALSE) -> ()  [unwired: 2 in, 2 out]
          }
        }
      }
    }
    n224 = case shown="True" "Open Device" {
      tunnel: [w208 w221] -> _
      tunnel: w27 -> [w208 _]
      tunnel: w30 -> [_ w220]
      tunnel: w28 -> [_ w212]
      tunnel: w29 -> [_ w211]
      frame False {
      }
      frame True {
        n225 = property on="Device List 2" class="Ring (strict)"() -> ("RingText.Text"=w210:string)  [unwired: 2 in, 2 out]
        n226 = String Subset(string=w210, offset (0)=1 ("偏移量(0)"), length (rest)=4 ("长度（剩余）")) -> (substring=w217:string)
        n227 = Equal?(x=w217, y="GigE") -> (x = y?=w216:bool)
        n228 = case shown="False" w216 {
          tunnel: [w230 w240] -> w225
          tunnel: [w229 w239] -> w209
          tunnel: w211 -> [w234 w242]
          tunnel: w220 -> [w231 w241]
          tunnel: w212 -> [w236 _]
          frame False {
            n229 = Array Size(array=w234) -> (size(s)=w233:i32)
            n230 = property on="Device List 2" class="Ring (strict)"() -> ("Value"=w235:u16)  [unwired: 2 in, 2 out]
            n231 = Subtract(x=w235, y=w233) -> (x-y=w232:i32)
            n232 = Index Array(array=w236, index=w232) -> (element=w228:T10)
            n233 = call-poly "CreateHandle.vi"("error in (no error)"=w231, "U3VDevice"=w228) -> ("error out"=w230:errorcluster, "handle"=w229:u64)  [unwired: 6 in, 1 out]
          }
          frame True {
            n234 = property on="Device List 2" class="Ring (strict)"() -> ("Value"=w237:u16)  [unwired: 2 in, 2 out]
            n235 = Index Array(array=w242, index=w237) -> (element=w238:T11)
            n236 = call-poly "CreateHandle.vi"("error in (no error)"=w241, "GigEDevice"=w238) -> ("error out"=w240:errorcluster, "handle"=w239:u64)  [unwired: 6 in, 1 out]
          }
        }
        "handle out 2" <- w209
        n237 = call "OpenDevice.vi"("error in (no error)"=w225, "nSwitchoverKey"=u16 0, "nAccessMode"=u32 1, "handle"=w209) -> ("error out"=w222:errorcluster, "return"=w214:i32, "handle out"=w213:u64)  [unwired: 5 in]
        n238 = Not Equal?(x=w214, y=0) -> (x != y?=w226:bool)
        n239 = case shown="False" w226 {
          tunnel: w213 -> [w243 w260]
          tunnel: w222 -> [w244 _]
          tunnel: [w243 u64 0 ("handle")] -> w221
          frame False {
            n240 = call "SetEnumValue.vi"("error in (no error)"=w244, "nValue"=u32 0, "strKey"="TriggerMode", "handle"=w243) -> ("error out"=w255:errorcluster)  [unwired: 5 in, 2 out]
            n241 = property on="Start" class="Bool"(error in=w255, "DisabledEnum"=T7."Enabled" ("禁用")) -> (error out=w253:errorcluster)  [unwired: 1 in, 1 out]
            n242 = property on="Open Device" class="Bool"(error in=w253, "DisabledEnum"=T7."Disabled and Grayed Out" ("禁用")) -> (error out=w252:errorcluster)  [unwired: 1 in, 1 out]
            n243 = property on="Close Device" class="Bool"(error in=w252, "DisabledEnum"=T7."Enabled" ("禁用")) -> (error out=w249:errorcluster)  [unwired: 1 in, 1 out]
            n244 = property on="Trigger Mode" class="Bool"(error in=w249, "DisabledEnum"=T7."Enabled" ("禁用")) -> (error out=w247:errorcluster)  [unwired: 1 in, 1 out]
            n245 = property on="Continuous" class="Bool"(error in=w247, "DisabledEnum"=T7."Disabled and Grayed Out" ("禁用")) -> (error out=w245:errorcluster)  [unwired: 1 in, 1 out]
            n246 = property on="打开标志" class="Bool (strict)"(error in=w245, "Value"=TRUE ("布尔")) -> ()  [unwired: 1 in, 2 out]
          }
          frame True {
            n247 = call "DestroyHandle.vi"("handle"=w260) -> ()  [unwired: 9 in, 2 out]
            n248 = One Button Dialog(message="Open Cam2 Failed") -> ()  [unwired: 1 in, 1 out]
            n249 = property on="打开标志" class="Bool (strict)"("Value"=FALSE) -> ()  [unwired: 2 in, 2 out]
          }
        }
      }
    }
    n250 = property on="handle out 2" class="DigNum (strict)"() -> ("Value"=w25:u64)  [unwired: 2 in, 2 out]
    n251 = case shown="True" "Close Device" {
      tunnel: w25 -> [_ w187]
      frame False {
      }
      frame True {
        n252 = call "CloseDevice.vi"("handle"=w187) -> ("error out"=w190:errorcluster, "handle out"=w188:u64)  [unwired: 8 in, 1 out]
        n253 = call "DestroyHandle.vi"("error in (no error)"=w190, "handle"=w188) -> ("error out"=w189:errorcluster)  [unwired: 8 in, 1 out]
        n254 = property on="Open Device" class="Bool"(error in=w189, "DisabledEnum"=T7."Enabled" ("禁用")) -> (error out=w203:errorcluster)  [unwired: 1 in, 1 out]
        n255 = property on="Close Device" class="Bool"(error in=w203, "DisabledEnum"=T7."Disabled and Grayed Out" ("禁用")) -> (error out=w202:errorcluster)  [unwired: 1 in, 1 out]
        n256 = property on="Start" class="Bool"(error in=w202, "DisabledEnum"=T7."Disabled and Grayed Out" ("禁用")) -> (error out=w201:errorcluster)  [unwired: 1 in, 1 out]
        n257 = property on="Stop" class="Bool"(error in=w201, "DisabledEnum"=T7."Disabled and Grayed Out" ("禁用")) -> (error out=w200:errorcluster)  [unwired: 1 in, 1 out]
        n258 = property on="Trigger Once" class="Bool"(error in=w200, "DisabledEnum"=T7."Disabled and Grayed Out" ("禁用")) -> (error out=w197:errorcluster)  [unwired: 1 in, 1 out]
        n259 = property on="Continuous" class="Bool"(error in=w197, "DisabledEnum"=T7."Disabled and Grayed Out" ("禁用")) -> (error out=w195:errorcluster)  [unwired: 1 in, 1 out]
        n260 = property on="Trigger Mode" class="Bool"(error in=w195, "DisabledEnum"=T7."Disabled and Grayed Out" ("禁用")) -> (error out=w194:errorcluster)  [unwired: 1 in, 1 out]
        n261 = property on="打开标志" class="Bool (strict)"(error in=w194, "Value"=FALSE ("打开标志")) -> (error out=w192:errorcluster)  [unwired: 1 in, 1 out]
        n262 = property on="Acquisision Flag" class="Bool (strict)"(error in=w192, "Value"=FALSE ("采集标志")) -> ()  [unwired: 1 in, 2 out]
      }
    }
    n263 = property on="handle out 2" class="DigNum (strict)"() -> ("Value"=w9:u64)  [unwired: 2 in, 2 out]
    n264 = property on="handle out" class="DigNum (strict)"() -> ("Value"=w43:u64)  [unwired: 2 in, 2 out]
  }
  n265 = property on="handle out" class="DigNum (strict)"() -> ("Value"=w3:u64)  [unwired: 2 in, 2 out]
  n266 = case shown="True" w5 {
    tunnel: w3 -> [_ w525]
    frame False {
    }
    frame True {
      n267 = property on="打开标志" class="Bool (strict)"() -> ("Value"=w516:bool)  [unwired: 2 in, 2 out]
      n268 = case shown="True" w516 {
        tunnel: w525 -> [_ w532]
        frame False {
        }
        frame True {
          n269 = call "CloseDevice.vi"("handle"=w532) -> ("error out"=w533:errorcluster, "handle out"=w531:u64)  [unwired: 8 in, 1 out]
          n270 = call "DestroyHandle.vi"("error in (no error)"=w533, "handle"=w531) -> ()  [unwired: 8 in, 2 out]
        }
      }
      n271 = property on="Open Device" class="Bool"("DisabledEnum"=T7."Enabled" ("禁用")) -> (error out=w524:errorcluster)  [unwired: 2 in, 1 out]
      n272 = property on="Close Device" class="Bool"(error in=w524, "DisabledEnum"=T7."Disabled and Grayed Out" ("禁用")) -> (error out=w523:errorcluster)  [unwired: 1 in, 1 out]
      n273 = property on="Trigger Once" class="Bool"(error in=w523, "DisabledEnum"=T7."Disabled and Grayed Out" ("禁用")) -> (error out=w522:errorcluster)  [unwired: 1 in, 1 out]
      n274 = property on="Start" class="Bool"(error in=w522, "DisabledEnum"=T7."Disabled and Grayed Out" ("禁用")) -> (error out=w521:errorcluster)  [unwired: 1 in, 1 out]
      n275 = property on="Stop" class="Bool"(error in=w521, "DisabledEnum"=T7."Disabled and Grayed Out" ("禁用")) -> (error out=w520:errorcluster)  [unwired: 1 in, 1 out]
      n276 = property on="Continuous" class="Bool"(error in=w520, "DisabledEnum"=T7."Disabled and Grayed Out" ("禁用")) -> (error out=w518:errorcluster)  [unwired: 1 in, 1 out]
      n277 = property on="Trigger Mode" class="Bool"(error in=w518, "DisabledEnum"=T7."Disabled and Grayed Out" ("禁用")) -> (error out=w513:errorcluster)  [unwired: 1 in, 1 out]
      n278 = property on="打开标志" class="Bool (strict)"(error in=w513, "Value"=FALSE ("打开标志")) -> (error out=w512:errorcluster)  [unwired: 1 in, 1 out]
      n279 = property on="Acquisision Flag" class="Bool (strict)"(error in=w512, "Value"=FALSE ("采集标志")) -> ()  [unwired: 1 in, 2 out]
    }
  }
  n280 = property on="handle out 2" class="DigNum (strict)"() -> ("Value"=w2:u64)  [unwired: 2 in, 2 out]
  n281 = case shown="True" w1 {
    tunnel: w2 -> [_ w547]
    frame False {
    }
    frame True {
      n282 = property on="打开标志" class="Bool (strict)"() -> ("Value"=w538:bool)  [unwired: 2 in, 2 out]
      n283 = case shown="True" w538 {
        tunnel: w547 -> [_ w554]
        frame False {
        }
        frame True {
          n284 = call "CloseDevice.vi"("handle"=w554) -> ("error out"=w555:errorcluster, "handle out"=w553:u64)  [unwired: 8 in, 1 out]
          n285 = call "DestroyHandle.vi"("error in (no error)"=w555, "handle"=w553) -> ()  [unwired: 8 in, 2 out]
        }
      }
      n286 = property on="Open Device" class="Bool"("DisabledEnum"=T7."Enabled" ("禁用")) -> (error out=w546:errorcluster)  [unwired: 2 in, 1 out]
      n287 = property on="Close Device" class="Bool"(error in=w546, "DisabledEnum"=T7."Disabled and Grayed Out" ("禁用")) -> (error out=w545:errorcluster)  [unwired: 1 in, 1 out]
      n288 = property on="Trigger Once" class="Bool"(error in=w545, "DisabledEnum"=T7."Disabled and Grayed Out" ("禁用")) -> (error out=w544:errorcluster)  [unwired: 1 in, 1 out]
      n289 = property on="Start" class="Bool"(error in=w544, "DisabledEnum"=T7."Disabled and Grayed Out" ("禁用")) -> (error out=w543:errorcluster)  [unwired: 1 in, 1 out]
      n290 = property on="Stop" class="Bool"(error in=w543, "DisabledEnum"=T7."Disabled and Grayed Out" ("禁用")) -> (error out=w542:errorcluster)  [unwired: 1 in, 1 out]
      n291 = property on="Continuous" class="Bool"(error in=w542, "DisabledEnum"=T7."Disabled and Grayed Out" ("禁用")) -> (error out=w540:errorcluster)  [unwired: 1 in, 1 out]
      n292 = property on="Trigger Mode" class="Bool"(error in=w540, "DisabledEnum"=T7."Disabled and Grayed Out" ("禁用")) -> (error out=w535:errorcluster)  [unwired: 1 in, 1 out]
      n293 = property on="打开标志" class="Bool (strict)"(error in=w535, "Value"=FALSE ("打开标志")) -> (error out=w534:errorcluster)  [unwired: 1 in, 1 out]
      n294 = property on="Acquisision Flag" class="Bool (strict)"(error in=w534, "Value"=FALSE ("采集标志")) -> ()  [unwired: 1 in, 2 out]
    }
  }
